vi "Cancel Current Operations.vi"(8 "error in (no error)":errorcluster, 11 "VISA resource name":refnum<visa-resource-name>) -> (0 "error out":errorcluster, 3 "VISA resource name out":refnum<visa-resource-name>)   [LabVIEW 2013, in "Watts Up Series.lvlib"]
doc: "Cancels all current data operations from the Watts Up meter."
uses:
  <instrlib>/Watts Up Series/Watts Up Series.lvlib
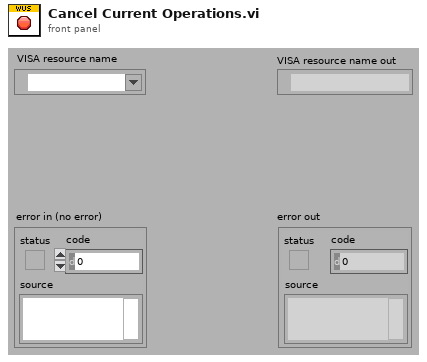
[diagram p1: front panel]
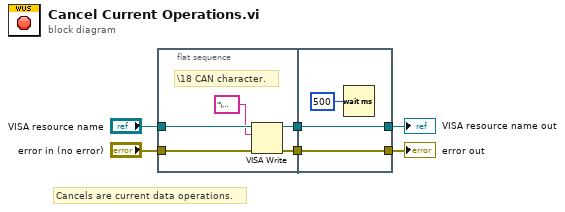
[diagram p0: block diagram]
diagram:
  # "Cancels are current data operations."
  n1 = flat-sequence {
    tunnel: "VISA resource name" -> [w11]
    tunnel: "error in (no error)" -> [w10]
    tunnel: [w9] -> w2
    tunnel: [w8] -> w1
    tunnel: [w13] -> w3
    tunnel: [w14] -> w4
    tunnel: w2 -> [w14]
    tunnel: w1 -> [w13]
    frame #0 {
      # "\\18 CAN character."
      n2 = VISA Write(VISA resource name=w11, write buffer="\u0018", error in (no error)=w10) -> (VISA resource name out=w9:refnum<visa-resource-name>, error out=w8:errorcluster)  [unwired: 1 out]
    }
    frame #1 {
      n3 = Wait (ms)(milliseconds to wait=u32 500) -> ()  [unwired: 1 out]
    }
  }
  "VISA resource name out" <- w4
  "error out" <- w3
